vi "verify WRITE SETUP parameters.vi"(8 "error in (no error)":errorcluster, 11 "Channel in":refnum<class "Channel.lvclass">) -> (0 "error out":errorcluster, 3 "Channel out":refnum<class "Channel.lvclass">)   [LabVIEW 2018, in "Channel.lvclass"]
uses:
  Channel.lvclass
  Channel.lvclass/Channel.ctl
  Simulated_CCD_Camera/Simulated Camera.lvclass/Simulated Camera.ctl
  Simulated_CCD_Camera/Simulated Camera.lvclass
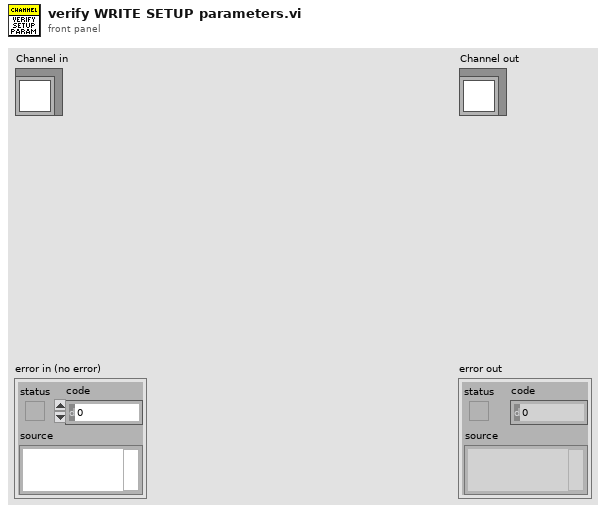
[diagram p1: front panel]
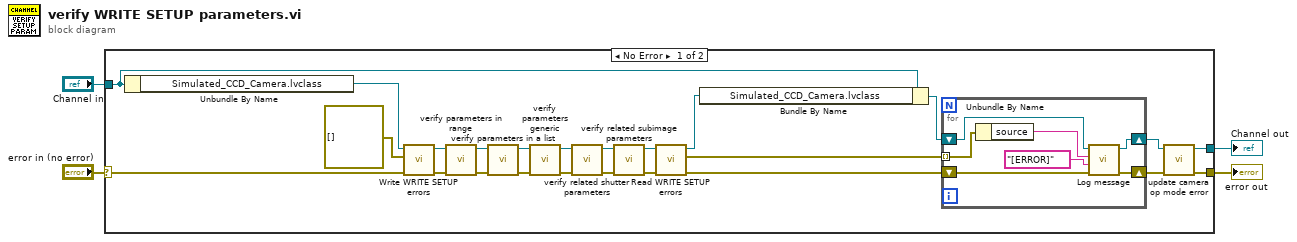
[diagram p0: block diagram]
diagram:
  n1 = case shown="No Error" "error in (no error)" {
    selector: "error in (no error)" -> [w17 w37]
    tunnel: [w13 w37] -> w3
    tunnel: [w14 w36] -> w1
    tunnel: "Channel in" -> [w28 w36]
    frame No Error {
      n2 = Unbundle By Name(w28) -> ("Simulated_CCD_Camera.lvclass"=w16:refnum<class "Simulated Camera.lvclass">)
      n3 = call "Write WRITE SETUP errors.vi"("error in (no error)"=w17, "WRITE SETUP errors"=errorcluster[] [] ("Errors array"), "Simulated_CCD_Camera in"=w16) -> ("error out"=w18:errorcluster, "Simulated_CCD_Camera out"=w19:refnum<class "Simulated Camera.lvclass">)  [unwired: 7 in]
      n4 = call "verify parameters in range.vi"("error in (no error)"=w18, "Simulated_CCD_Camera in"=w19) -> ("error out"=w27:errorcluster, "Simulated_CCD_Camera out"=w26:refnum<class "Simulated Camera.lvclass">)  [unwired: 8 in]
      n5 = call "verify parameters in a list.vi"("error in (no error)"=w27, "Simulated_CCD_Camera in"=w26) -> ("error out"=w20:errorcluster, "Simulated_CCD_Camera out"=w21:refnum<class "Simulated Camera.lvclass">)  [unwired: 8 in]
      n6 = call "verify parameters generic.vi"("error in (no error)"=w20, "Simulated_CCD_Camera in"=w21) -> ("error out"=w22:errorcluster, "Simulated_CCD_Camera out"=w23:refnum<class "Simulated Camera.lvclass">)  [unwired: 8 in]
      n7 = call "verify related shutter parameters.vi"("error in (no error)"=w22, "Simulated_CCD_Camera in"=w23) -> ("error out"=w24:errorcluster, "Simulated_CCD_Camera out"=w25:refnum<class "Simulated Camera.lvclass">)  [unwired: 8 in]
      n8 = call "verify related subimage parameters.vi"("error in (no error)"=w24, "Simulated_CCD_Camera in"=w25) -> ("error out"=w9:errorcluster, "Simulated_CCD_Camera out"=w10:refnum<class "Simulated Camera.lvclass">)  [unwired: 8 in]
      n9 = call "Read WRITE SETUP errors.vi"("error in (no error)"=w9, "Simulated_CCD_Camera in"=w10) -> ("error out"=w12:errorcluster, "WRITE SETUP errors"=w11:errorcluster[], "Simulated_CCD_Camera out"=w5:refnum<class "Simulated Camera.lvclass">)  [unwired: 7 in]
      n10 = Bundle By Name(cluster=w28, "Simulated_CCD_Camera.lvclass"=w5) -> (w7:refnum<class "Channel.lvclass">)
      n11 = for {
        shift-right: [w34] -> w6
        shift-left: w7 -> [w35]
        shift-right: [w33] -> w8
        shift-left: w12 -> [w31]
        tunnel: w11 -> [w30] mode=indexing
        n12 = Unbundle By Name(w30) -> ("source"=w29:string)
        n13 = call "Log message.vi"("error in (no error)"=w31, "message type"="[ERROR]", "String"=w29, "Channel in"=w35) -> ("error out"=w33:errorcluster, "Channel out"=w34:refnum<class "Channel.lvclass">)  [unwired: 6 in]
      }
      n14 = call "update camera op mode error.vi"("error in (no error)"=w8, "Channel in"=w6) -> ("error out"=w13:errorcluster, "Channel out"=w14:refnum<class "Channel.lvclass">)  [unwired: 8 in]
    }
    frame Error {
    }
  }
  "error out" <- w3
  "Channel out" <- w1
